vi "Nd array string check.vi"() -> ()   [LabVIEW 2013]
uses:
  JSONtext.lvlib
panel:
  out "3d flat/unflat jtxt->lvj pok":bool
  out "3d flat/unflat jtxt->lvj":errorcluster
  out "3d lvjson match jsontxt":bool
  out "3d err (does not throw err)":errorcluster
  out "3d ok (not supported right now)":bool
  out "1d err":errorcluster
  out "1d ok":bool
  out "2d ok":bool
  out "2d err":errorcluster
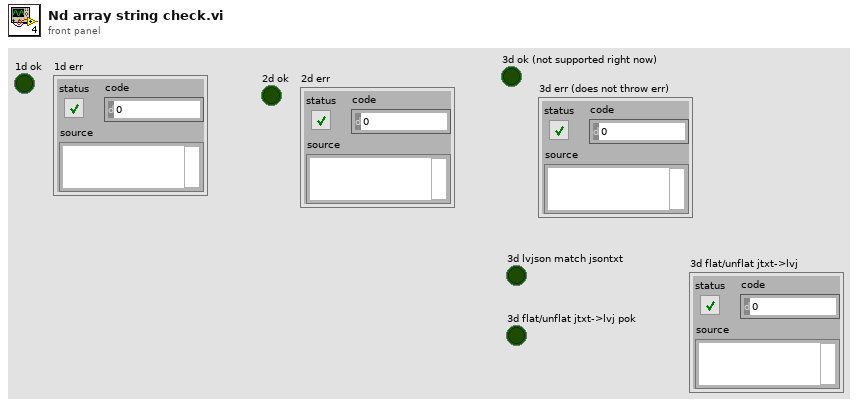
[diagram p1: front panel]
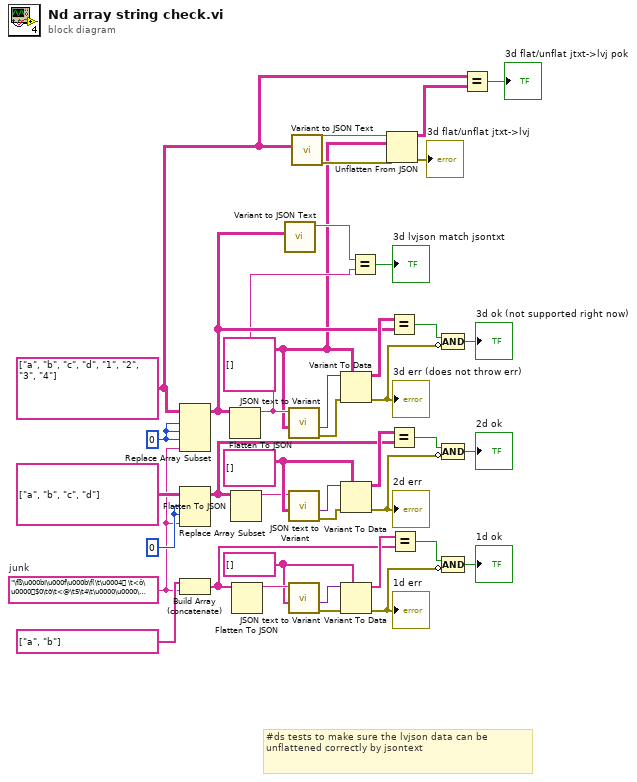
[diagram p0: block diagram]
diagram:
  w13 = 0 ("index (page)")
  w14 = 0 ("disabled index (col)")
  w12 = "\fß\u000bI\u000f\u000b\f(\t\u0004 \t<ô\u0000$0\tð\t<@\t5\t4\t\u0000\u0000\u0000\u0000\u0000\u0000\u0000ïï2\b\t2\u0000í÷\b> x\u0003ô\f\t#\u0004\r\u0001\b\u0012\u0001-\n!3\u0001\u0002\u0003\u0004\u0005\u0006\u0007\b\t\u0010\n\u000b\f\r\u000e\u000f\u0001\u0001\u0011!1AQaq¡±ÁÑ"  # junk
  w18 = string[] [] ("<JSON> 2")
  w19 = string[][] [] ("<JSON> 2")
  w5 = string[][][] [] ("<JSON> 2")
  w1 = string[][][] [[["a", "b"], ["c", "d"]], [["1", "2"], ["3", "4"]]] ("Array")
  # "#ds tests to make sure the lvjson data can be unflattened correctly by jsontext"
  n1 = Replace Array Subset(array=w1, new element=w12, index (dim 0)=w13, index (dim 1)=w13, index (dim 2)=w13) -> (w11:string[][][])
  n2 = Replace Array Subset(array=string[][] [["a", "b"], ["c", "d"]] ("Array"), new element=w12, index (row)=w14, index (col)=w14) -> (w15:string[][])
  n3 = Build Array (concatenate)(string[] ["a", "b"] ("Array"), w12) -> (w16:string[])
  n4 = Flatten To JSON(anything=w11) -> (JSON string=w10:string)  [unwired: 2 in, 1 out]
  n5 = Flatten To JSON(anything=w15) -> (JSON string=w17:string)  [unwired: 2 in, 1 out]
  n6 = Flatten To JSON(anything=w16) -> (JSON string=w20:string)  [unwired: 2 in, 1 out]
  n7 = call "Variant to JSON Text.vi"("Variant"=w11) -> ("<JSON>"=w9:string)  [unwired: 9 in, 1 out]
  n8 = call "JSON text to Variant.vi"("Data Type"=w5, "JSON"=w10) -> ("error out"=w36:errorcluster, "Variant out"=w35:variant)  [unwired: 8 in]
  n9 = call "JSON text to Variant.vi"("Data Type"=w19, "JSON"=w17) -> ("error out"=w33:errorcluster, "Variant out"=w34:variant)  [unwired: 8 in]
  n10 = call "JSON text to Variant.vi"("Data Type"=w18, "JSON"=w20) -> ("error out"=w22:errorcluster, "Variant out"=w21:variant)  [unwired: 8 in]
  n11 = call "Variant to JSON Text.vi"("Variant"=w1) -> ("error out"=w7:errorcluster, "<JSON>"=w6:string)  [unwired: 9 in]
  n12 = Variant To Data(error in=w36, type=w5, Variant=w35) -> (data=w38:string[][][], error out=w37:errorcluster)
  "3d err (does not throw err)" <- w37
  n13 = Variant To Data(error in=w33, type=w19, Variant=w34) -> (data=w31:string[][], error out=w32:errorcluster)
  "2d err" <- w32
  n14 = Variant To Data(error in=w22, type=w18, Variant=w21) -> (data=w24:string[], error out=w23:errorcluster)
  "1d err" <- w23
  n15 = Equal?(x=w9, y=w10) -> (x = y?=→"3d lvjson match jsontxt":bool)
  n16 = Unflatten From JSON(JSON string=w6, type and defaults=w5, error in (no error)=w7) -> (value=w3:string[][][], error out=→"3d flat/unflat jtxt->lvj":errorcluster)  [unwired: 4 in]
  n17 = Equal?(x=w38, y=w11) -> (x = y?=w39:bool)
  n18 = Equal?(x=w31, y=w15) -> (x = y?=w29:bool)
  n19 = Equal?(x=w24, y=w16) -> (x = y?=w26:bool)
  n20 = Compound Arithmetic op=AND(w39, invert w37) -> (→"3d ok (not supported right now)":bool)
  n21 = Compound Arithmetic op=AND(w29, invert w32) -> (→"2d ok":bool)
  n22 = Compound Arithmetic op=AND(w26, invert w23) -> (→"1d ok":bool)
  n23 = Equal?(x=w1, y=w3) -> (x = y?=→"3d flat/unflat jtxt->lvj pok":bool)
